vi "Read_Electrical_Variables.vi"(8 "error in (no error)":errorcluster, 11 "Modbus master in":refnum<class "Modbus Master.lvclass">) -> (0 "error out":errorcluster, 2 "Variables":sgl[](array[numeric]), 3 "Modbus master out":refnum<class "Modbus Master.lvclass">)   [LabVIEW 2017]
uses:
  <vilib>/Modbus/master/Modbus Master.lvclass
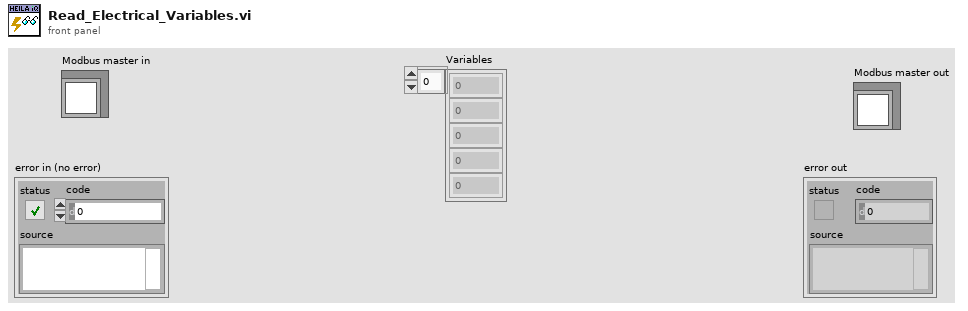
[diagram p1: front panel]
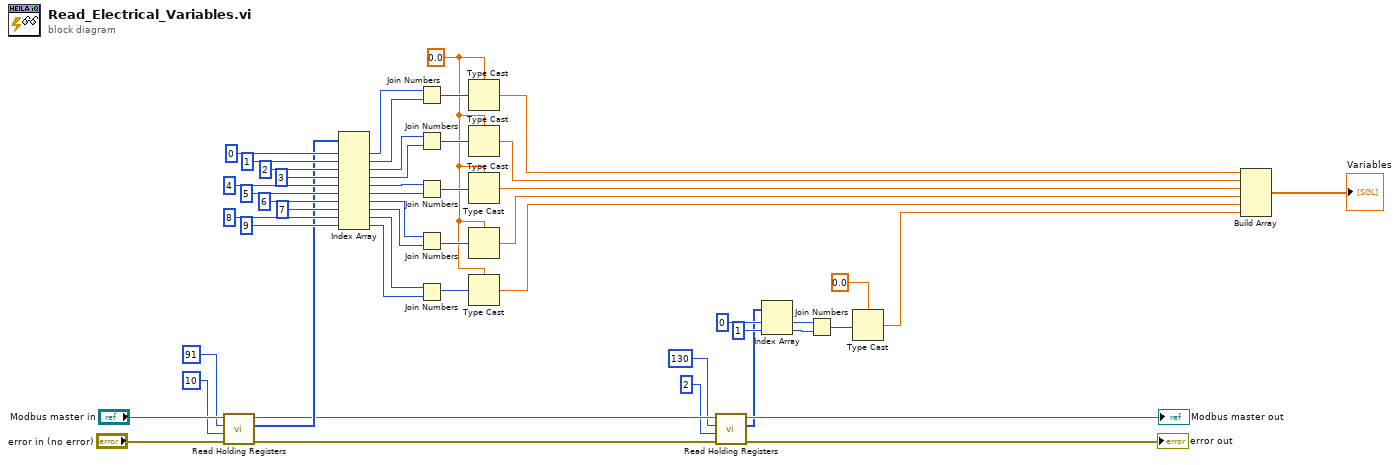
[diagram p0: block diagram]
diagram:
  w21 = sgl 0.0
  n1 = call-dynamic "Read Holding Registers.vi"("error in (no error)"="error in (no error)", "number of holding registers"=u16 10 ("starting address"), "starting address"=u16 91, "Modbus master in"="Modbus master in") -> ("error out"=w13:errorcluster, "register values"=w36:u16[], "Modbus master out"=w14:refnum<class "Modbus Master.lvclass">)  [unwired: 5 in]
  n2 = Index Array(array=w36, index #1=0 ("index"), index #2=1 ("index"), index #3=2 ("index"), index #4=3 ("index"), index #5=4 ("index"), index #6=5 ("index"), index #7=6 ("index"), index #8=7 ("index"), index #9=8 ("index"), index #10=9 ("index")) -> (element #1=w37:u16, element #2=w35:u16, element #3=w34:u16, element #4=w33:u16, element #5=w32:u16, element #6=w31:u16, element #7=w30:u16, element #8=w29:u16, element #9=w28:u16, element #10=w27:u16)
  n3 = Join Numbers(hi=w37, lo=w35) -> ((hi.lo)=w26:u32)
  n4 = Join Numbers(hi=w34, lo=w33) -> ((hi.lo)=w25:u32)
  n5 = Join Numbers(hi=w32, lo=w31) -> ((hi.lo)=w24:u32)
  n6 = Join Numbers(hi=w30, lo=w29) -> ((hi.lo)=w23:u32)
  n7 = Join Numbers(hi=w28, lo=w27) -> ((hi.lo)=w22:u32)
  n8 = Type Cast(type=w21, x=w26) -> (*(type *) &x=w20:sgl)
  n9 = Type Cast(type=w21, x=w25) -> (*(type *) &x=w19:sgl)
  n10 = Type Cast(type=w21, x=w24) -> (*(type *) &x=w18:sgl)
  n11 = Type Cast(type=w21, x=w23) -> (*(type *) &x=w17:sgl)
  n12 = Type Cast(type=w21, x=w22) -> (*(type *) &x=w16:sgl)
  n13 = call-dynamic "Read Holding Registers.vi"("error in (no error)"=w13, "number of holding registers"=u16 2 ("starting address"), "starting address"=u16 130, "Modbus master in"=w14) -> ("error out"=→"error out":errorcluster, "register values"=w6:u16[], "Modbus master out"=→"Modbus master out":refnum<class "Modbus Master.lvclass">)  [unwired: 5 in]
  n14 = Index Array(array=w6, index #1=0 ("index"), index #2=1 ("index")) -> (element #1=w5:u16, element #2=w4:u16)
  n15 = Join Numbers(hi=w5, lo=w4) -> ((hi.lo)=w3:u32)
  n16 = Type Cast(type=sgl 0.0, x=w3) -> (*(type *) &x=w1:sgl)
  n17 = Build Array(w20, w19, w18, w17, w16, w1) -> (→"Variables":sgl[])
